vi "RasterScan-CentroidSelectionGUI.vi"(5 "Raster Scan":dbl[][](graph), 7 "X":dbl[][](array[numeric]), 9 "Y":dbl[][](array[numeric]), 12 "X in":dbl, 14 "Y in":dbl) -> (1 "X out":dbl, 3 "Y out":dbl)   [LabVIEW 2009]
panel:
  in  "CANCEL Button":bool
  in  "MAXIMUM Button":bool
  in  "BARYCENTER Button":bool
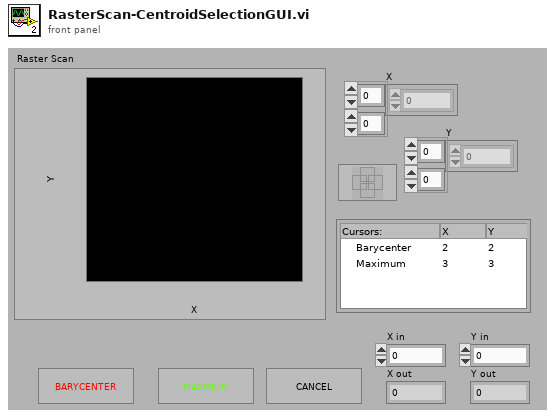
[diagram p1: front panel]
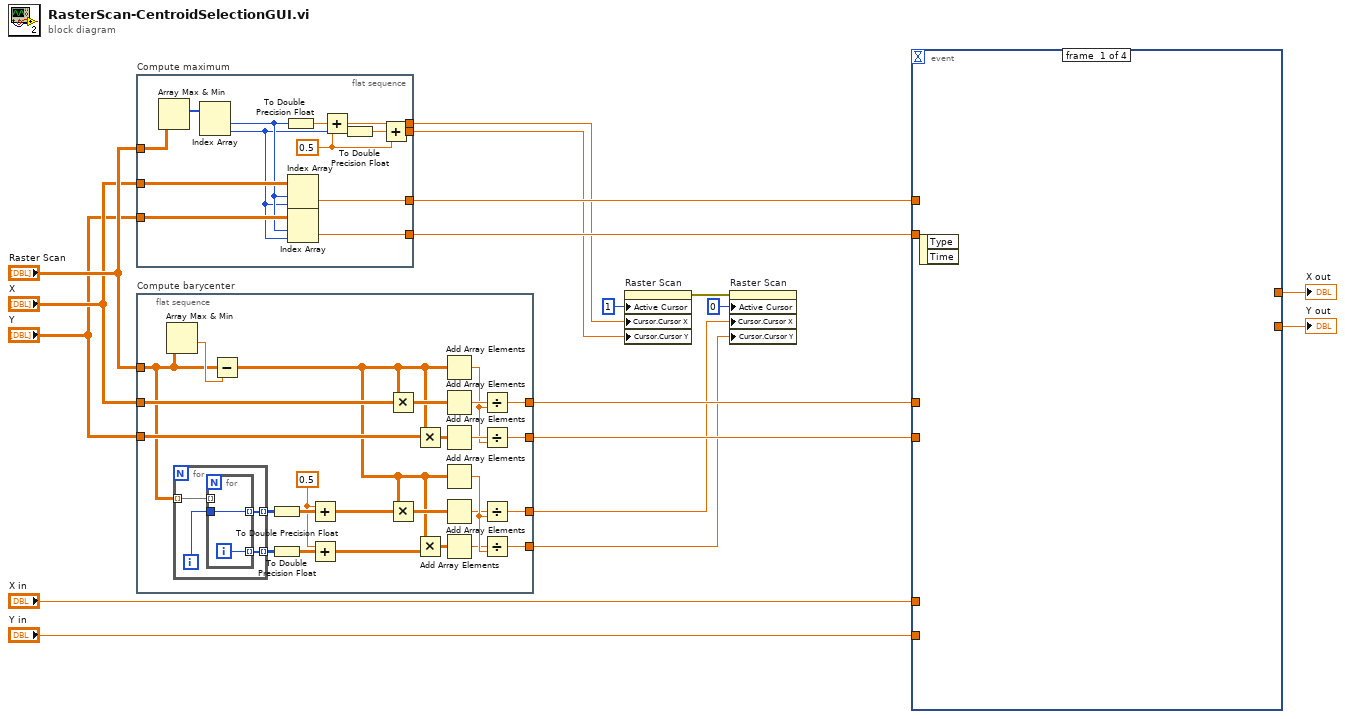
[diagram p0: block diagram]
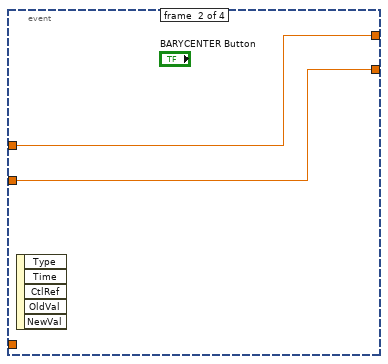
[diagram p2: hidden frame]
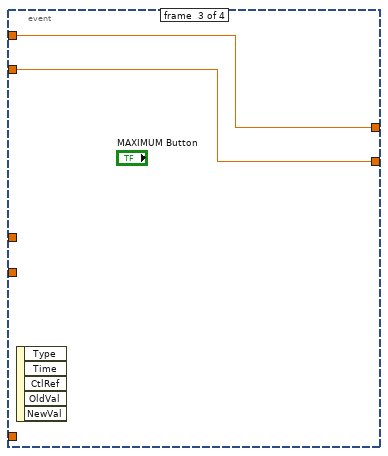
[diagram p3: hidden frame]
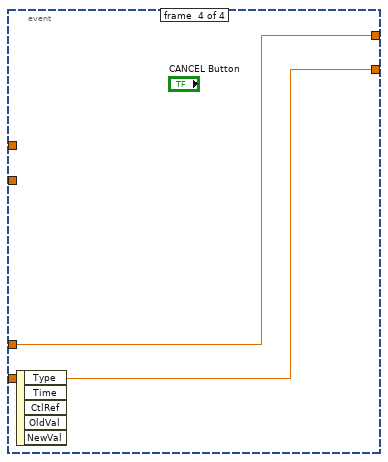
[diagram p4: hidden frame]
diagram:
  n1 = flat-sequence "Compute maximum" {
    tunnel: "X" -> [w29]
    tunnel: "Y" -> [w28]
    tunnel: "Raster Scan" -> [w31]
    tunnel: [w27] -> w15
    tunnel: [w26] -> w14
    tunnel: [w20] -> w6
    tunnel: [w19] -> w5
    frame #0 {
      w21 = 0.5 ("y")
      n2 = Array Max & Min(array=w31) -> (max index (indices)=w30:i32[])  [unwired: 3 out]
      n3 = Index Array(array=w30) -> (element #1=w25:i32, element #2=w22:i32)  [unwired: 2 in]
      n4 = To Double Precision Float(number=w25) -> (double precision float=w24:dbl)
      n5 = Index Array(array=w29, index (row)=w25, index (col)=w22) -> (element=w27:dbl)
      n6 = Index Array(array=w28, index (row)=w25, index (col)=w22) -> (element=w26:dbl)
      n7 = Add(x=w24, y=w21) -> (x+y=w20:dbl)
      n8 = To Double Precision Float(number=w22) -> (double precision float=w23:dbl)
      n9 = Add(x=w23, y=w21) -> (x+y=w19:dbl)
    }
  }
  n10 = flat-sequence "Compute barycenter" {
    tunnel: "X" -> [w57]
    tunnel: "Y" -> [w56]
    tunnel: "Raster Scan" -> [w47]
    tunnel: [w49] -> w13
    tunnel: [w48] -> w12
    tunnel: [w33] -> w2
    tunnel: [w32] -> w1
    frame #0 {
      w42 = 0.5 ("y")
      n11 = Array Max & Min(array=w47) -> (min value=w50:dbl)  [unwired: 3 out]
      n12 = for {
        tunnel: w47 -> [w61] mode=indexing
        tunnel: [w59] -> w46 mode=indexing
        tunnel: [w58] -> w45 mode=indexing
        i -> [w60]
        n13 = for {
          tunnel: w61 -> [_] mode=indexing
          tunnel: w60 -> [w62]
          tunnel: [w63] -> w58 mode=indexing
          tunnel: [w62] -> w59 mode=indexing
          i -> [w63]
        }
      }
      n14 = Subtract(x=w47, y=w50) -> (x-y=w36:dbl[][])
      n15 = To Double Precision Float(number=w46) -> (double precision float=w44:dbl[][])
      n16 = To Double Precision Float(number=w45) -> (double precision float=w43:dbl[][])
      n17 = Add(x=w42, y=w44) -> (x+y=w35:dbl[][])
      n18 = Add(x=w42, y=w43) -> (x+y=w34:dbl[][])
      n19 = Multiply(x=w36, y=w57) -> (x*y=w55:dbl[][])
      n20 = Multiply(x=w36, y=w35) -> (x*y=w37:dbl[][])
      n21 = Multiply(x=w36, y=w56) -> (x*y=w54:dbl[][])
      n22 = Multiply(x=w36, y=w34) -> (x*y=w38:dbl[][])
      n23 = Add Array Elements(numeric array=w36) -> (sum=w51:dbl)
      n24 = Add Array Elements(numeric array=w55) -> (sum=w53:dbl)
      n25 = Add Array Elements(numeric array=w54) -> (sum=w52:dbl)
      n26 = Add Array Elements(numeric array=w36) -> (sum=w41:dbl)
      n27 = Add Array Elements(numeric array=w37) -> (sum=w39:dbl)
      n28 = Add Array Elements(numeric array=w38) -> (sum=w40:dbl)
      n29 = Divide(x=w53, y=w51) -> (x/y=w49:dbl)
      n30 = Divide(x=w52, y=w51) -> (x/y=w48:dbl)
      n31 = Divide(x=w39, y=w41) -> (x/y=w33:dbl)
      n32 = Divide(x=w40, y=w41) -> (x/y=w32:dbl)
    }
  }
  n33 = property on="Raster Scan" class="IntGraph (strict)"("Active Cursor"=u32 1, "Cursor.Cursor X"=w6, "Cursor.Cursor Y"=w5) -> (error out=w3:errorcluster)  [unwired: 2 in, 1 out]
  n34 = property on="Raster Scan" class="IntGraph (strict)"(error in=w3, "Active Cursor"=u32 0, "Cursor.Cursor X"=w2, "Cursor.Cursor Y"=w1) -> ()  [unwired: 1 in, 2 out]
  n35 = event shown="[3] \"CANCEL Button\": Value Change" {
    selector: _ -> [_ _ _ _]
    dyn-events: _ -> [_ _ _ _]
    timeout: _ -> [_ _ _ _]
    tunnel: w15 -> [_ _ w67 _]
    tunnel: w14 -> [_ _ w66 _]
    tunnel: w13 -> [_ w65 _ _]
    tunnel: w12 -> [_ w64 _ _]
    tunnel: "X in" -> [_ _ _ w69]
    tunnel: "Y in" -> [_ _ _ w68]
    tunnel: [_ w65 w67 w69] -> w9
    tunnel: [_ w64 w66 w68] -> w8
    event #0 {
      n36 = event-data() -> ()  [unwired: 1 in, 2 out]
    }
    event #1 {
      n37 = event-data() -> ()  [unwired: 1 in, 5 out]
    }
    event #2 {
      n38 = event-data() -> ()  [unwired: 1 in, 5 out]
    }
    event #3 {
      n39 = event-data() -> ()  [unwired: 1 in, 5 out]
    }
  }
  "X out" <- w9
  "Y out" <- w8
